vi "Node Has Roles.vi"(8 "error in (no error)":errorcluster, 11 "VolatusAPI in":refnum<class "VolatusAPI.lvclass">) -> (0 "error out":errorcluster, 2 "Node Has Roles":bool, 3 "VolatusAPI out":refnum<class "VolatusAPI.lvclass">)   [LabVIEW 2020, in "Volatus.lvlib" / "VolatusAPI.lvclass"]
uses:
  VolatusAPI.lvclass
  VolatusAPI.lvclass/VolatusAPI.ctl
  VolatusConfig/VolatusConfigElement/VolatusConfigElement.lvclass
  lv-cdm/CDM-Config/Config Filter/Config Lookup.lvclass
  VolatusConfig/VolatusConfig.lvlib
  VolatusConfig/Meta Type.ctl
  VolatusConfig/Node/Node Config.lvclass
  C:/dev/lv20CE/relink/lv-volatus/VolatusConfig/VolatusConfigElement/VolatusConfigElement.lvclass
  C:/dev/lv20CE/relink/lv-volatus/VolatusConfig/Node/Node Config.lvclass
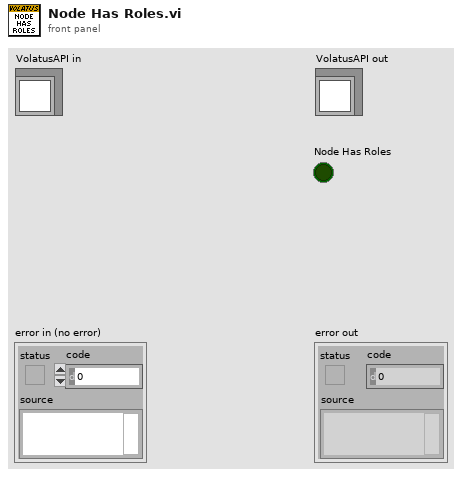
[diagram p1: front panel]
types:
  T1 = typedef "VolatusConfig.lvlib/Meta Type.ctl" = enum16{"UNKNOWN", "VL_System", "VL_Cluster", "VL_Node", "VL_Task", "VL_Group", "VL_Channel", "VL_Task_List", "VL_Scaling", "VL_Sensor", "VL_Sensor_List", "VL_Scale"}
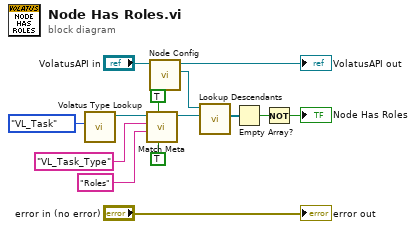
[diagram p0: block diagram]
diagram:
  n1 = call "Volatus Type Lookup.vi"("Meta Type"=Meta_Type."VL_Task") -> ("Config Lookup out"=w4:refnum<class "Config Lookup.lvclass">)  [unwired: 9 in, 1 out]
  n2 = call "Match Meta.vi"("Exact Value (F)"=TRUE, "Don't Recurse Past Match"=TRUE, "Value (Any)"="Roles" ("Name"), "Name"="VL_Task_Type", "Config Lookup (New)"=w4) -> ("Config Lookup out"=w9:refnum<class "Config Lookup.lvclass">)  [unwired: 5 in, 1 out]
  n3 = call "Node Config.vi"("VolatusAPI in"="VolatusAPI in") -> ("Node Config"=w8:refnum<class "Node Config.lvclass">, "VolatusAPI out"=→"VolatusAPI out":refnum<class "VolatusAPI.lvclass">)  [unwired: 9 in]
  n4 = call "Lookup Descendants.vi"("Lookup"=w9, "VolatusConfigElement in"=w8) -> ("Descendants"=w7:refnum<class "Config Element.lvclass">[])  [unwired: 7 in, 2 out]
  n5 = Empty Array?(array=w7) -> (empty?=w6:bool)
  n6 = Not(x=w6) -> (.not. x?=→"Node Has Roles":bool)
  "error out" <- "error in (no error)"
